vi "Complex Vector x A.vi"(2 "Matrix A":T1, 3 "Vector V'":cdb[](array[numeric])) -> (0 "error":i32, 1 "V' x A":cdb[](array[numeric]))   [LabVIEW 2018, in "NI_AALBase.lvlib"]
doc: "Performs the multiplication of two input matrices or an input matrix and an input vector. The data types you wire to the <B>A</B> and <B>B</B> inputs determine the polymorphic instance to use."
uses:
  NI_AALBase.lvlib
  ComplexMatrix.ctl
  <resource>/lvanlys.dll
  NI_Matrix.lvlib
panel:
  # "Complex Vector x A"
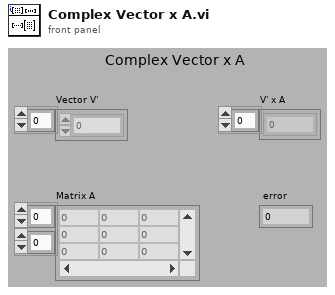
[diagram p1: front panel]
types:
  T1 = typedef "NI_Matrix.lvlib/ComplexMatrix.ctl" = cdb[][]
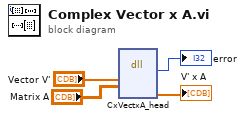
[diagram p0: block diagram]
diagram:
  n1 = dll-call lib="C:/Program Files (x86)/National Instruments/LabVIEW 2018/resource/lvanlys.*" fn="CxVectxA_head"("Vector V'"="Vector V'", "Matrix A"="Matrix A") -> (→"error":i32, "V' x A"=→"V' x A":cdb[])  [unwired: 6 in, 2 out]
